vi "list and create PG AI table 64.vi"(8 "error in":errorcluster, 9 "AI table":string[](array[string]), 10 "table name":string, 11 "conn":u64) -> (0 "error out":errorcluster, 3 "conn_out":u64)   [LabVIEW 2019, in "PostgreSQL.lvlib"]
uses:
  PostgreSQL.lvlib
  PostgreSQL2LabVIEW/libpqlv64/src/PQresultErrorMessage.vi
  PostgreSQL2LabVIEW/libpqUtility64/src/PQclear.vi
  PostgreSQL2LabVIEW/libpqlv64/src/PQsendQuery.vi
  PostgreSQL2LabVIEW/libpqlv64/src/PQgetResult.vi
  PostgreSQL2LabVIEW/libpqlv64/src/PQresultStatus.vi
  PostgreSQL2LabVIEW/libpqUtility64/src/PQgetColumn.vi
  PostgreSQL2LabVIEW/libpqlv64/src/PQclear.vi
  PostgreSQL2LabVIEW/libpqUtility64/src/PQfetchTables.vi
  PostgreSQL2LabVIEW/libpqlv64/src/PQgetvalue.vi
  PostgreSQL2LabVIEW/libpqlv64/src/PQntuples.vi
  PostgreSQL2LabVIEW/libpqUtility64/libpqutility64.lvlib
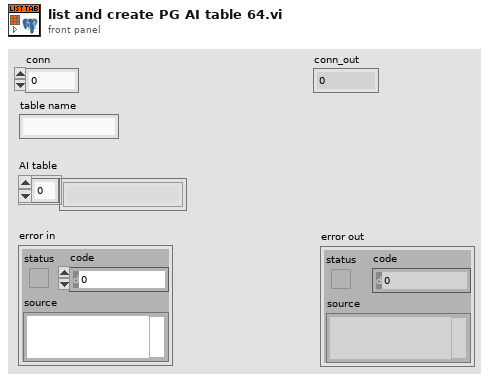
[diagram p1: front panel]
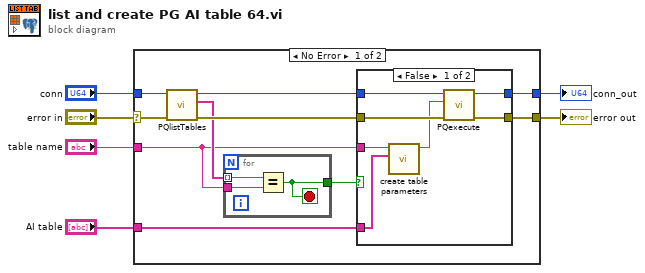
[diagram p0: block diagram]
diagram:
  n1 = case shown="No Error" "error in" {
    selector: "error in" -> [w13 w30]
    tunnel: "conn" -> [w10 w29]
    tunnel: [w16 w29] -> w4
    tunnel: "AI table" -> [w7 _]
    tunnel: [w15 w30] -> w3
    tunnel: "table name" -> [w8 _]
    frame No Error {
      n2 = call "PQlistTables.vi"("error in"=w13, "conn"=w10) -> ("error out"=w12:errorcluster, "Data"=w9:string[], "conn_out"=w11:u64)  [unwired: 7 in]
      n3 = for {
        tunnel: w8 -> [w18]
        tunnel: w9 -> [w19] mode=indexing
        tunnel: [w17] -> w14
        stop <- w17 stop-if-true
        n4 = Equal?(x=w19, y=w18) -> (x = y?=w17:bool)
      }
      n5 = case shown="False" w14 {
        tunnel: w11 -> [w24 w28]
        tunnel: [w21 w28] -> w16
        tunnel: w12 -> [w23 w27]
        tunnel: [w20 w27] -> w15
        tunnel: w7 -> [w25 _]
        tunnel: w8 -> [w26 _]
        frame False {
          n6 = call "create table parameters.vi"("AI table"=w25, "table name"=w26) -> ("create table parameters"=w22:string)  [unwired: 9 in]
          n7 = call "PQexecute.vi"("error in"=w23, "SQL querry"=w22, "conn"=w24) -> ("error out"=w20:errorcluster, "conn_out"=w21:u64)  [unwired: 7 in]
        }
        frame True {
        }
      }
    }
    frame Error {
    }
  }
  "conn_out" <- w4
  "error out" <- w3
